vi "Get Fast Axis Parameters.vi"(8 "error in (no error)":errorcluster, 11 "Galvo in":refnum<class "Galvo.lvclass">) -> (0 "error out":errorcluster, 2 "Fast Axis Parameters":T1, 3 "Galvo out":refnum<class "Galvo.lvclass">)   [LabVIEW 2015, in "Galvo.lvclass"]
uses:
  Galvo.lvclass
  Fast Axis Parameters.ctl
  Galvo.lvclass/Galvo.ctl
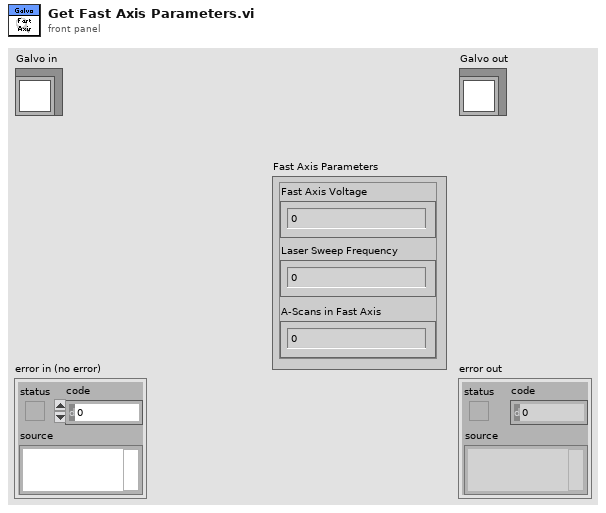
[diagram p1: front panel]
types:
  T1 = typedef "Galvo.lvclass/Fast Axis Parameters.ctl" = cluster{"Fast Axis Voltage":dbl, "Laser Sweep Frequency":dbl, "A-Scans in Fast Axis":dbl}
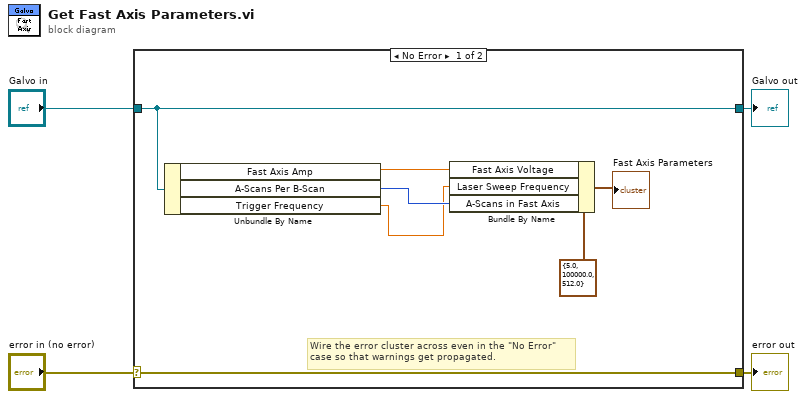
[diagram p0: block diagram]
diagram:
  n1 = case shown="No Error" "error in (no error)" {
    selector: "error in (no error)" -> [w11 w13]
    tunnel: [w11 w13] -> w3
    tunnel: [w10 w12] -> w1
    tunnel: "Galvo in" -> [w10 w12]
    frame No Error {
      # "Wire the error cluster across even in the \"No Error\"\ncase so that warnings get propagated."
      n2 = Unbundle By Name(w10) -> ("Fast Axis Amp"=w5:sgl, "A-Scans Per B-Scan"=w7:u32, "Trigger Frequency"=w6:dbl)
      n3 = Bundle By Name(cluster=T1 {"Fast Axis Voltage"=5.0, "Laser Sweep Frequency"=100000.0, "A-Scans in Fast Axis"=512.0} ("Fast Axis Parameters 2"), "Fast Axis Voltage"=w5, "Laser Sweep Frequency"=w6, "A-Scans in Fast Axis"=w7) -> (→"Fast Axis Parameters":T1)
    }
    frame Error {
    }
  }
  "error out" <- w3
  "Galvo out" <- w1
